vi "GetJSONFromVI.vi"() -> ()   [LabVIEW 2019, in "LabJSON.lvlib"]
doc: "Get all controls/indicators of a VI as JSON"
uses:
  LabJSON.lvlib
  <vilib>/SLL Toolkit/SLL File IO/SLL File IO.lvlib
panel:
  in  "Controls?":bool=TRUE
  in  "Error In":errorcluster
  out "Error Out":errorcluster
  out "JSON Output":string
  in  "VI Path":path=path "Sample/SampleVI.vi"
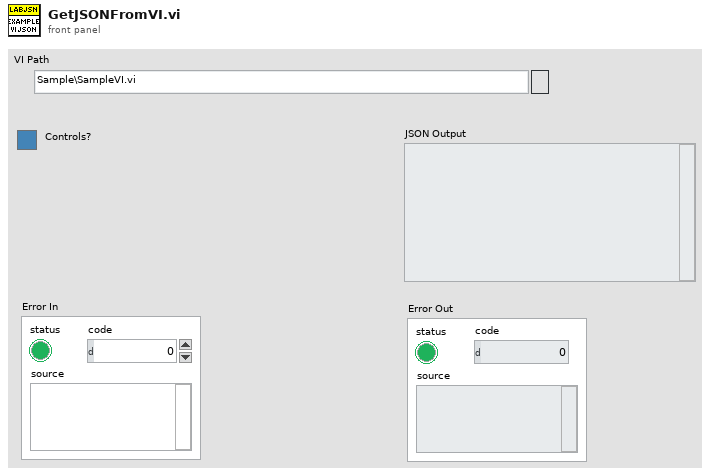
[diagram p1: front panel]
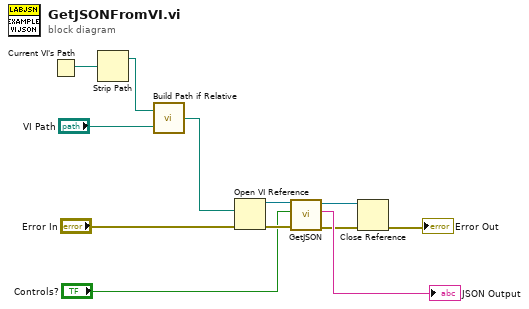
[diagram p0: block diagram]
diagram:
  n1 = Current VI's Path() -> (path=w11:path)
  n2 = Strip Path(path=w11) -> (stripped path=w10:path)  [unwired: 1 out]
  n3 = call <vilib>:"Build Path if Relative.vi"("Relative or Absolute Path"="VI Path", "Base Path"=w10) -> ("Path Out"=w8:path)
  n4 = Open VI Reference(vi path=w8, error in (no error)="Error In") -> (vi reference=w6:refnum<vi>, error out=w7:errorcluster)  [unwired: 4 in]
  n5 = call "GetJSON.vi"("Error In"=w7, "Controls?"="Controls?", "VI Refnum In"=w6) -> ("Error Out"=w3:errorcluster, "JSON Out"=→"JSON Output":string, "VI Refnum Out"=w1:refnum<vi>)  [unwired: 6 in]
  n6 = Close Reference(reference=w1, error in (no error)=w3) -> (error out=→"Error Out":errorcluster)
